vi "boolean to radio button.vi"(1 "Boolean":bool) -> (0 "Radio Buttons":enum32{"Radio Selection 1", "Radio Selection 2"}(radio))   [LabVIEW 2019]
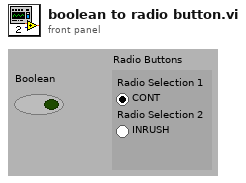
[diagram p1: front panel]
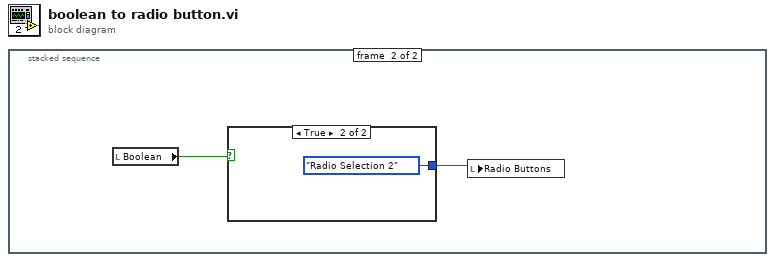
[diagram p0: block diagram]
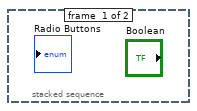
[diagram p2: hidden frame]
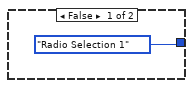
[diagram p3: hidden frame]
diagram:
  n1 = stacked-sequence {
    frame #0 {
    }
    frame #1 {
      n2 = local read "Boolean"() -> (w2:bool)
      n3 = case shown="True" w2 {
        tunnel: [enum32{"Radio Selection 1", "Radio Selection 2"}."Radio Selection 1" ("Radio Buttons") enum32{"Radio Selection 1", "Radio Selection 2"}."Radio Selection 2" ("Radio Buttons")] -> w1
        frame False {
        }
        frame True {
        }
      }
      n4 = local write "Radio Buttons"(w1) -> ()
    }
  }
